vi "UnpackFieldsFromAny.vi"(8 "error in":errorcluster, 11 "Any":T1) -> (0 "error out":errorcluster, 3 "Fields Ref Out":T2)   [LabVIEW 2019, in "gprc-lvsupport.lvlib"]
uses:
  gprc-lvsupport.lvlib
  typeDefs/grpcId.ctl
  typeDefs/Any.ctl
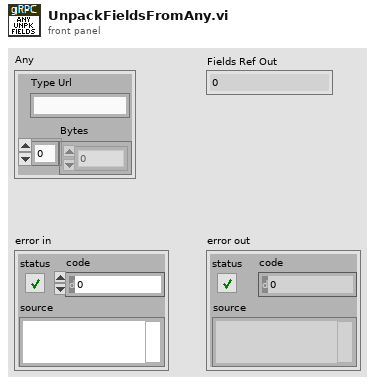
[diagram p1: front panel]
types:
  T1 = typedef "gprc-lvsupport.lvlib/Any.ctl" = cluster{"Type Url":string, "Bytes":u8[]}
  T2 = typedef "gprc-lvsupport.lvlib/grpcId.ctl" = u64
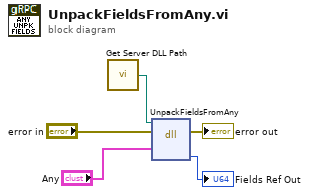
[diagram p0: block diagram]
diagram:
  n1 = call "Get Server DLL Path.vi"() -> ("Server dll path"=w3:path)
  n2 = dll-call lib="?" fn="UnpackFieldsFromAny"(path in=w3, error in="error in", "any"="Any") -> (error out=→"error out":errorcluster, "elementRef"=→"Fields Ref Out":u64)  [unwired: 4 in, 1 out]
